vi "Wait For CLIP Ready.vi"(0 "Refnum in":refnum<k20>, 11 "error in":errorcluster) -> (4 "Refnum out":refnum<k20>, 6 "sFrontEndConfig_Complete":bool, 15 "error out":errorcluster)   [LabVIEW 2016, in "Aurora Stream (NI 6592R) (Host).lvlib"]
doc: "Waits until the CLIP has finished self-configuration (indicated by <b>sFrontEndConfig_Complete</b> and both Port0_UserClk and Port2_UserClk are up and running.\n\n<B>Input Parameters</B>\n\n<B>Refnum in</B> Receives a reference to the FPGA from the previous VI.\n\n<B>error in</B> describes error conditions that occur before this node runs. This input provides standard error in functionality.\n\n<B>Output Parameters</B>\n\n<B>Refnum out</B> passes a reference to the FPGA to the next VI.\n\n<B>sFrontEndConfig_Complete</B> is True if the FPGA's front end configuration has completed.\n\n<B>error out</B> contains error information. This output provides standard error out functionality."
uses:
  Aurora Stream (NI 6592R) (Host).lvlib
  <vilib>/Utility/error.llb/Error Cluster From Error Code.vi
  <vilib>/rvi/errors/niLvFpgaAdjustHostInterfaceError.vi
  <vilib>/rvi/interface/nirviReadWriteControl/nirviReadWriteControl.xnode
  NiFpgaLv.dll
  <vilib>/rvi/interface/Simulation/niFpgaSimulationCallBeginRW.vi
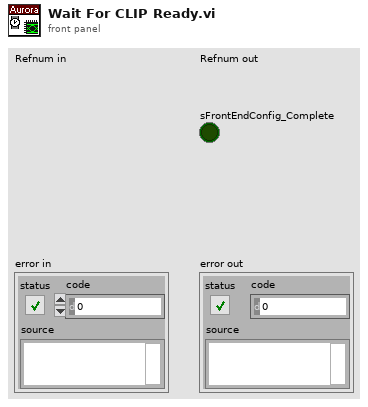
[diagram p1: front panel]
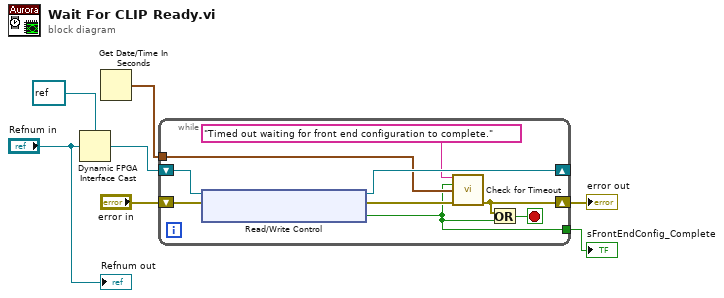
[diagram p0: block diagram]
diagram:
  n1 = Dynamic FPGA Interface Cast(Session In=refnum<k20> refnum ("FPGA Interface"), Type="Refnum in") -> (Session Out=w2:refnum<k20>)
  n2 = Get Date/Time In Seconds() -> (seconds since 1Jan1904=w7:timestamp)
  n3 = while {
    shift-right: [w13] -> _
    shift-left: w2 -> [w15]
    shift-right: [w11] -> w5
    shift-left: "error in" -> [w14]
    tunnel: w7 -> [w10]
    tunnel: [w8] -> w4
    stop <- w16 stop-if-true
    n4 = xnode "Read/Write Control"("FPGA VI Reference In"=w15, "error in"=w14) -> ("FPGA VI Reference Out"=w13:refnum<k20>, "error out"=w12:errorcluster, "sFrontEndConfig_Complete"=w8:bool)
    n5 = call "Check for Timeout.vi"("Error Message"="Timed out waiting for front end configuration to complete." ("error message (\"\")"), "Complete?"=w8, "Start Time"=w10, "error in"=w12) -> ("error out"=w11:errorcluster)  [unwired: 11 in]
    n6 = Or(x=w11, y=w8) -> (x .or. y?=w16:bool)
  }
  "error out" <- w5
  "sFrontEndConfig_Complete" <- w4
  "Refnum out" <- "Refnum in"
